vi "NML Analog Display.vi"() -> ()   [LabVIEW 2021]
doc: "Continuous display of M input channels averaged over N readings and scaled by an offset and multiplicatve factor.\nScott Hannahs, NHMFL, July 2021\n<sth@magnet.fsu.edu>"
uses:
  <vilib>/Utility/error.llb/DialogType.ctl
  <vilib>/_DAQmxBase/Internals/DAQmxBase Create Channel (AI-Voltage-Basic).vi
  <vilib>/_DAQmxBase/Internals/DAQmxBase Timing (Sample Clock).vi
  <vilib>/_DAQmxBase/Internals/DAQmxBase Read (Analog 2D DBL NChan NSamp).vi
panel:
  out "Scaled Values":dbl[](array[numeric]) caption="Scaled Measurement" format="%.5f"
  in  "Scale":dbl[](array[numeric])=[0.0, 20.0, 20.0, 4.3, 5.15, 1.0, 1.0, 1.0, 1.0, 1.0, 1.0, 1.0, 1.0, 1.0, 1.0, 1.0] format="%.5f"
  in  "Offset":dbl[](array[numeric])=[0.0, 0.0, 0.0, -2.0, -2.0, 0.0, 0.0, 0.0, 0.0, 0.0, 0.0, 0.0, 0.0, 0.0, 0.0, 0.0] format="%.5f"
  out "Scan Backlog":u32
  out "Display Iteration":i32
  out "Acq Iteration":i32
  in  "Physical Channel":tag="Dev1/ai0:7,Dev1/ai16:23"
  in  "Samples to Read":i32=1000
  in  "Minimum Value":dbl=-10.0 format="%0.2f"
  in  "Maximum Value":dbl=10.0 format="%0.2f"
  in  "stop":bool
  in  "Sample Rate":dbl=4000.0 caption="Sample Rate (Hz)"
  out "Raw Voltage":dbl[](array[numeric]) caption="Raw Measurement" format="%.5f"
  # "For instructions, select Help>>Show Context Help"
  # "Channel Parameters"
  # "Timing Parameters"
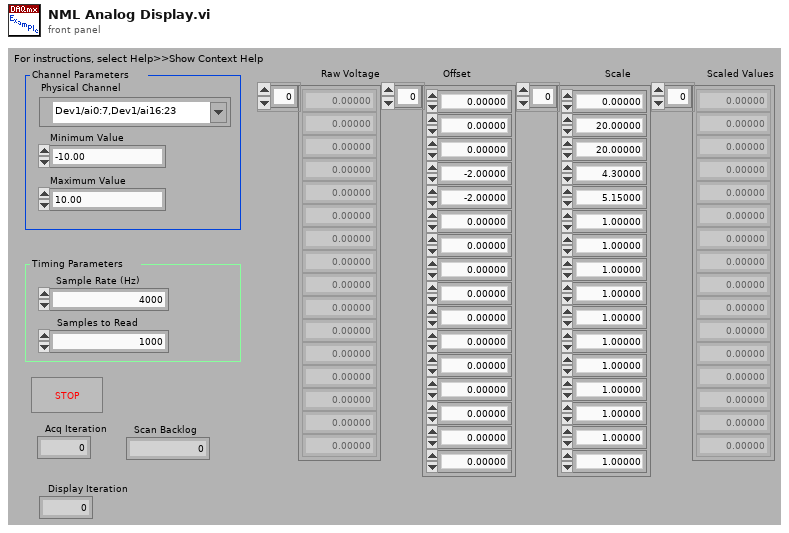
[diagram p1: front panel]
types:
  T1 = typedef "DialogType.ctl" = u16
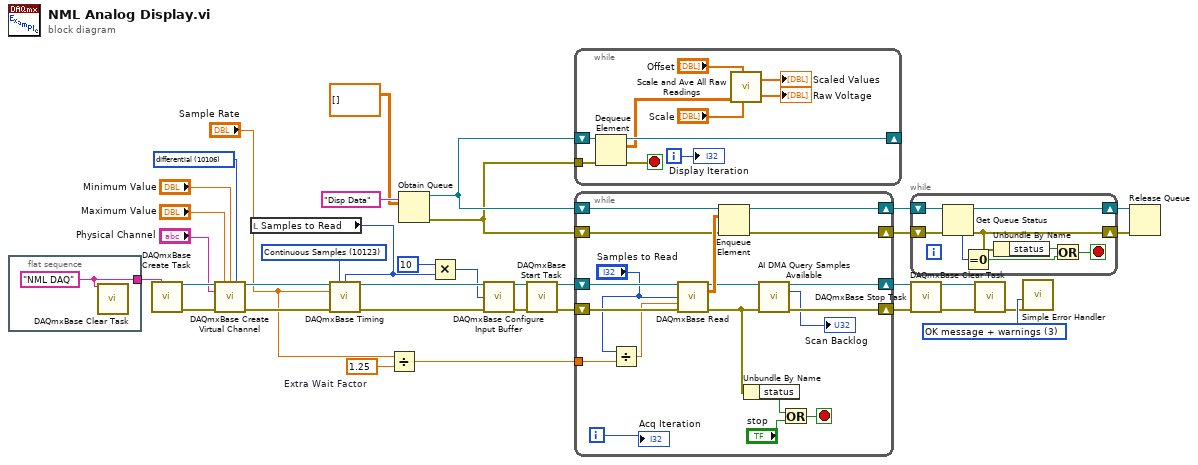
[diagram p0: block diagram]
diagram:
  w1 = 1.25  # Extra Wait Factor
  w18 = 10106 items=["default"=-1, "differential"=10106, "RSE"=10083, "NRSE"=10078] ("input terminal configuration")
  w35 = T1 3 items=["no dialog", "OK message", "continue or stop message", "OK message + warnings", "continue/stop + warnings"] ("type of dialog (OK msg:1)")
  w22 = 10123 items=["Finite Samples"=10178, "Continuous Samples"=10123] ("sample mode")
  n1 = flat-sequence {
    tunnel: [w36] -> w8
    frame #0 {
      w36 = "NML DAQ" ("new task name")
      n2 = call <vilib>:"DAQmxBase Clear Task.vi"("task in"=w36) -> ()  [unwired: 14 in, 1 out]
    }
  }
  n3 = call <vilib>:"DAQmxBase Create Task.vi"("new task name"=w8) -> ("task out"=w33:refnum<k21>, "error out"=w34:errorcluster)  [unwired: 13 in]
  n4 = call-poly <vilib>:"DAQmxBase Create Virtual Channel.vi"("task in"=w33, "maximum value"="Maximum Value", "minimum value"="Minimum Value", "input terminal configuration"=w18, "physical channels"="Physical Channel", "error in"=w34) -> ("task out"=w31:refnum<k21>, "error out"=w32:errorcluster)  [unwired: 8 in]
  n5 = local read "Samples to Read"() -> (w6:i32)
  n6 = call-poly <vilib>:"DAQmxBase Timing.vi"("task/channels in"=w31, "sample mode"=w22, "samples per channel"=w6, "rate"="Sample Rate", "error in"=w32) -> ("task out"=w29:refnum<k21>, "error out"=w30:errorcluster)  [unwired: 9 in]
  n7 = Divide(x="Sample Rate", y=w1) -> (x/y=w2:dbl)
  n8 = Obtain Queue(name (unnamed)="Disp Data", element data type=dbl[][] [] ("data")) -> (queue out=w10:refnum<queue>, error out=w9:errorcluster)  [unwired: 3 in, 1 out]
  n9 = Multiply(x=u32 10, y=w6) -> (x*y=w5:u32)
  n10 = call <vilib>:"DAQmxBase Configure Input Buffer.vi"("task/channels in"=w29, "buffer size (in samples per channel)"=w5) -> ("task out"=w7:refnum<k21>)  [unwired: 12 in, 1 out]
  n11 = call <vilib>:"DAQmxBase Start Task.vi"("task/channels in"=w7, "error in"=w30) -> ("task out"=w28:refnum<k21>, "error out"=w16:errorcluster)  [unwired: 12 in]
  n12 = while {
    shift-right: [w45] -> _
    shift-left: w10 -> [w46]
    tunnel: w9 -> [w42]
    i -> [w41]
    stop <- w43 stop-if-true
    n13 = Dequeue Element(queue=w46, error in (no error)=w42) -> (queue out=w45:refnum<queue>, element=w44:dbl[][], error out=w43:errorcluster)  [unwired: 1 in, 1 out]
    n14 = call "Scale and Ave All Raw Readings.vi"("Scale"="Scale", "Offset"="Offset", "Input Array"=w44) -> ("Raw Voltage"=→"Raw Voltage":dbl[], "Scaled Array"=→"Scaled Values":dbl[])  [unwired: 3 in]
    "Display Iteration" <- w41
  }
  n15 = while {
    shift-right: [w56] -> w12
    shift-left: w9 -> [w55]
    shift-right: [w57] -> w13
    shift-left: w10 -> [w58]
    tunnel: w2 -> [w47]
    shift-right: [w52] -> w27
    shift-left: w28 -> [w64]
    shift-right: [w53] -> w23
    shift-left: w16 -> [w65]
    i -> [w60]
    stop <- w61 stop-if-true
    n16 = Divide(x="Samples to Read", y=w47) -> (x/y=w49:dbl)
    n17 = call-poly <vilib>:"DAQmxBase Read.vi"("task/channels in"=w64, "number of samples per channel"="Samples to Read", "timeout"=w49, "error in"=w65) -> ("task out"=w51:refnum<k21>, "data"=w59:dbl[][], "error out"=w54:errorcluster)  [unwired: 9 in]
    n18 = Enqueue Element(queue=w58, element=w59, error in (no error)=w55) -> (queue out=w57:refnum<queue>, error out=w56:errorcluster)  [unwired: 1 in, 1 out]
    n19 = Unbundle By Name(w54) -> ("status"=w62:bool)
    n20 = call "AI DMA Query Samples Available.vi"("task in"=w51, "error in"=w54) -> ("task out"=w52:refnum<k21>, "samples per chan available"=→"Scan Backlog":u32, "error out"=w53:errorcluster)  [unwired: 11 in]
    n21 = Or(x=w62, y="stop") -> (x .or. y?=w61:bool)
    "Acq Iteration" <- w60
  }
  n22 = while {
    shift-right: [w69] -> w14
    shift-left: w12 -> [w72]
    shift-right: [w71] -> w15
    shift-left: w13 -> [w73]
    stop <- w70 stop-if-true
    n23 = Get Queue Status(queue=w73, error in (no error)=w72) -> (queue out=w71:refnum<queue>, error out=w69:errorcluster, # elements in queue=w68:i32)  [unwired: 1 in, 5 out]
    n24 = Equal To 0?(x=w68) -> (x = 0?=w66:bool)
    n25 = Unbundle By Name(w69) -> ("status"=w67:bool)
    n26 = Or(x=w67, y=w66) -> (x .or. y?=w70:bool)
  }
  n27 = call <vilib>:"DAQmxBase Stop Task.vi"("task/channels in"=w27, "error in"=w23) -> ("task out"=w25:refnum<k21>, "error out"=w26:errorcluster)  [unwired: 12 in]
  n28 = call <vilib>:"DAQmxBase Clear Task.vi"("task in"=w25, "error in"=w26) -> ("error out"=w24:errorcluster)  [unwired: 13 in]
  n29 = call <vilib>:"Simple Error Handler.vi"("type of dialog (OK msg:1)"=w35, "error in (no error)"=w24) -> ()  [unwired: 3 in, 5 out]
  n30 = Release Queue(queue=w15, error in (no error)=w14) -> ()  [unwired: 1 in, 3 out]
